vi "LoadIOLabel.vi"(8 "error in":errorcluster, 11 "file path":path) -> (0 "error out":errorcluster, 2 "OutputLabel":string[](array[string]), 3 "InputLabel":string[](array[string]))   [LabVIEW 2015]
uses:
  <vilib>/Utility/config.llb/Read Key (String).vi
  <vilib>/Utility/config.llb/NI_LVConfig.lvlib
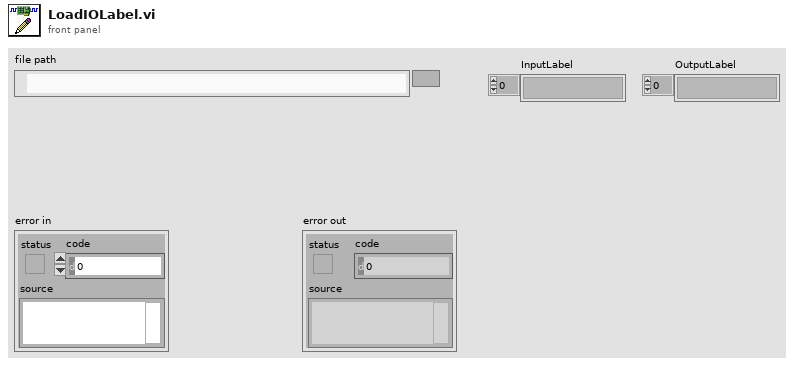
[diagram p1: front panel]
types:
  T1 = typedef "NI_LVConfig.lvlib/Config Data RefNum.ctl" = refnum<k1>
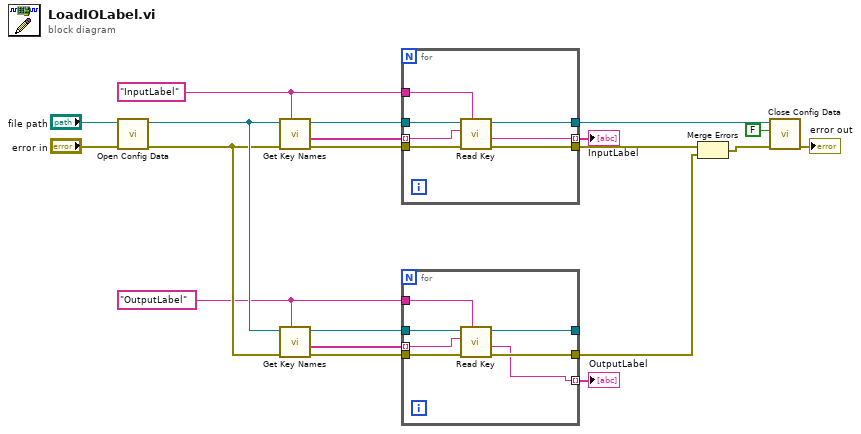
[diagram p0: block diagram]
diagram:
  w10 = "OutputLabel" ("section")
  w13 = "InputLabel" ("section")
  n1 = call <vilib>:"Open Config Data.vi"("error in (no error)"="error in", "configuration file path"="file path") -> ("error out"=w17:errorcluster, "refnum"=w18:T1)  [unwired: 7 in, 1 out]
  n2 = call <vilib>:"Get Key Names.vi"("section"=w13, "error in (no error)"=w17, "refnum"=w18) -> ("error out"=w14:errorcluster, "key names"=w16:string[], "refnum out"=w15:T1)  [unwired: 5 in, 1 out]
  n3 = call <vilib>:"Get Key Names.vi"("section"=w10, "error in (no error)"=w17, "refnum"=w18) -> ("error out"=w9:errorcluster, "key names"=w8:string[], "refnum out"=w11:T1)  [unwired: 5 in, 1 out]
  n4 = for {
    tunnel: w16 -> [w27] mode=indexing
    tunnel: w15 -> [w26]
    tunnel: w14 -> [w25]
    tunnel: w13 -> [w24]
    tunnel: [w21] -> w2 mode=indexing
    tunnel: [w23] -> w7
    tunnel: [w22] -> w12
    n5 = call-poly <vilib>:"Read Key.vi"("section"=w24, "error in (no error)"=w25, "key"=w27, "refnum"=w26) -> ("error out"=w23:errorcluster, "value"=w21:string, "refnum out"=w22:T1)  [unwired: 4 in, 1 out]
  }
  "InputLabel" <- w2
  n6 = for {
    tunnel: w8 -> [w34] mode=indexing
    tunnel: w11 -> [w33]
    tunnel: w9 -> [w32]
    tunnel: w10 -> [w31]
    tunnel: [w30] -> w6
    tunnel: [w29] -> _
    tunnel: [w28] -> w1 mode=indexing
    n7 = call-poly <vilib>:"Read Key.vi"("section"=w31, "error in (no error)"=w32, "key"=w34, "refnum"=w33) -> ("error out"=w30:errorcluster, "value"=w28:string, "refnum out"=w29:T1)  [unwired: 4 in, 1 out]
  }
  "OutputLabel" <- w1
  n8 = Merge Errors(w7, w6) -> (w5:errorcluster)
  n9 = call <vilib>:"Close Config Data.vi"("error in (no error)"=w5, "write file if changed (T)"=FALSE, "refnum"=w12) -> ("error out"=→"error out":errorcluster)  [unwired: 7 in, 1 out]
